vi "Butterfly_extract_VPI_VRL - LHL CFree Offset.vi"(8 "C_Free":dbl[](array[numeric]), 9 "Delta":dbl, 10 "Voltage Array":dbl[](array[numeric]), 11 "Result Array In":dbl[][](array[numeric])) -> (2 "VRLs":dbl[](array[numeric]), 3 "VPIs":dbl[](array[numeric]))   [LabVIEW 2013]
doc: "Extracts the VPI and VRL with respect to the given threshold for a data set that starts low value, goes above threshold, and comes back below the threshold (LHL)."
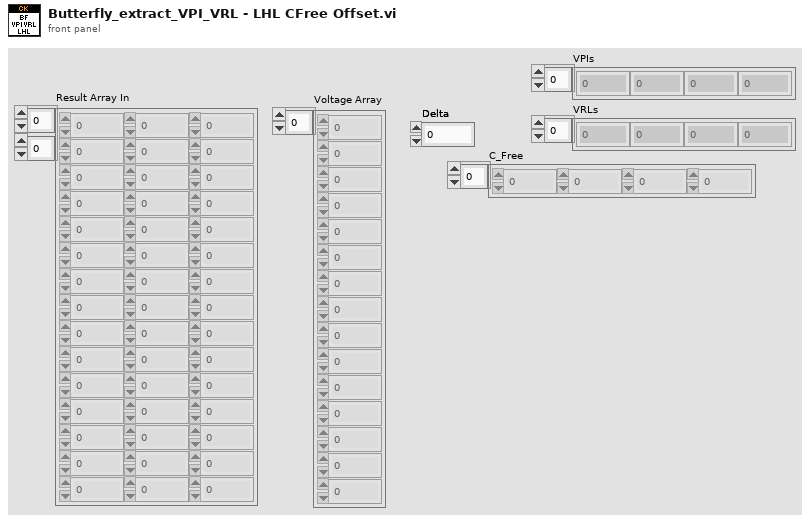
[diagram p1: front panel]
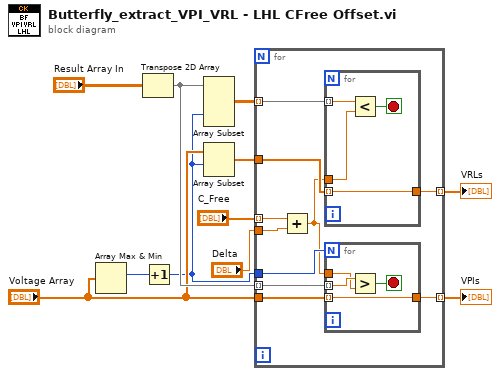
[diagram p0: block diagram]
diagram:
  n1 = Array Max & Min(array="Voltage Array") -> (max index (indices)=w9:i32)  [unwired: 3 out]
  n2 = Transpose 2D Array(2D array="Result Array In") -> (transposed array=w5:dbl[][])
  n3 = Increment(x=w9) -> (x+1=w2:i32)
  n4 = Array Subset(array=w5, index (col)=w2) -> (w8:dbl[][])  [unwired: 3 in]
  n5 = Array Subset(array="Voltage Array", index=w2) -> (w4:dbl[])  [unwired: 1 in]
  n6 = for {
    tunnel: w5 -> [w17] mode=indexing
    tunnel: "Delta" -> [w14]
    tunnel: [w21] -> w10 mode=indexing
    tunnel: w2 -> [w16]
    tunnel: "Voltage Array" -> [w19]
    tunnel: w8 -> [w20] mode=indexing
    tunnel: [w18] -> w7 mode=indexing
    tunnel: w4 -> [w15]
    tunnel: "C_Free" -> [w13] mode=indexing
    n7 = Add(x=w13, y=w14) -> (x+y=w12:dbl)
    n8 = for {
      tunnel: w20 -> [w25] mode=indexing
      tunnel: w12 -> [w24]
      tunnel: w15 -> [w22] mode=indexing
      tunnel: [w22] -> w18
      stop <- w23 stop-if-true
      n9 = Less?(x=w25, y=w24) -> (x < y?=w23:bool)
    }
    n10 = for {
      N: w16 -> [_]
      tunnel: w17 -> [w29] mode=indexing
      tunnel: w12 -> [w28]
      tunnel: w19 -> [w26] mode=indexing
      tunnel: [w26] -> w21
      stop <- w27 stop-if-true
      n11 = Greater?(x=w29, y=w28) -> (0:w27:bool)
    }
  }
  "VPIs" <- w10
  "VRLs" <- w7
